vi "ObtainQueue.vi"() -> (0 "error out":errorcluster, 1 "LowLevelQue":refnum<queue>, 2 "SequenceQue":refnum<queue>, 3 "EventQue":refnum<queue>)   [LabVIEW 2017]
uses:
  Event clusterr.ctl
  EventMsg.ctl
  Sequence cluster.ctl
  SequenceMsg.ctl
  LowLevel cluster.ctl
  LowLevelMsg.ctl
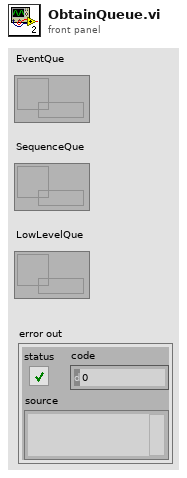
[diagram p1: front panel]
types:
  T1 = typedef "LowLevel cluster.ctl" = cluster{"LowLevelMsg":T2, "LowLevel string":string}
  T2 = typedef "LowLevelMsg.ctl" = enum16{"ResetArduinoState", "Init", "Halt", "SetArduinoState", "RunStopSigGen", "Error"}
  T3 = typedef "Sequence cluster.ctl" = cluster{"SequenceMsg":T4, "Sequence String":string}
  T4 = typedef "SequenceMsg.ctl" = enum16{"Init", "Halt", "Load", "RunStop", "Back", "NextManual", "NextSequenceStep", "Reset"}
  T5 = typedef "Event clusterr.ctl" = cluster{"EventMsg":T6, "Event string":string}
  T6 = typedef "EventMsg.ctl" = enum16{"Init", "Halt", "Listen"}
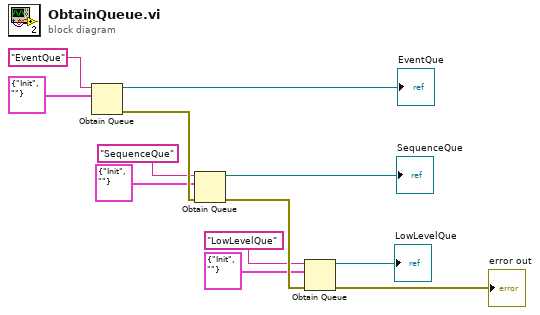
[diagram p0: block diagram]
diagram:
  n1 = Obtain Queue(name (unnamed)="EventQue", element data type=T5 {"EventMsg"=enum."Init", "Event string"=""} ("Event cluster")) -> (queue out=→"EventQue":refnum<queue>, error out=w6:errorcluster)  [unwired: 3 in, 1 out]
  n2 = Obtain Queue(name (unnamed)="SequenceQue", element data type=T3 {"SequenceMsg"=enum."Init", "Sequence String"=""} ("Sequence Cluster"), error in (no error)=w6) -> (queue out=→"SequenceQue":refnum<queue>, error out=w9:errorcluster)  [unwired: 2 in, 1 out]
  n3 = Obtain Queue(name (unnamed)="LowLevelQue", element data type=T1 {"LowLevelMsg"=enum."Init", "LowLevel string"=""} ("LowLevel cluster"), error in (no error)=w9) -> (queue out=→"LowLevelQue":refnum<queue>, error out=→"error out":errorcluster)  [unwired: 2 in, 1 out]
